vi "Test - Serial Device - Write Pin 1.vi"(8 "error in (no error)":errorcluster, 11 "Module ID":i32) -> (0 "error out":errorcluster, 3 "Pass":bool)   [LabVIEW 2020]
doc: "_____\nCreated using Delacor QMH Event Scripter 5.0.0.112."
uses:
  Libraries/Serial Device/Serial Device.lvlib
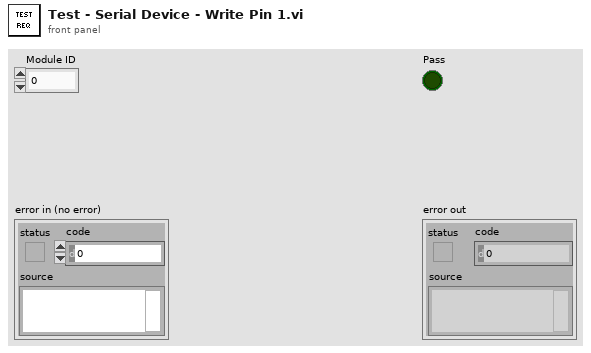
[diagram p1: front panel]
types:
  T1 = typedef "Serial Device.lvlib/Broadcast Events--cluster.ctl" = cluster{"Module Did Init":refnum<user-event>, "Status Updated":refnum<user-event>, "Error Reported":refnum<user-event>, "Module Did Stop":refnum<user-event>, "Update Module Execution Status":refnum<user-event>}
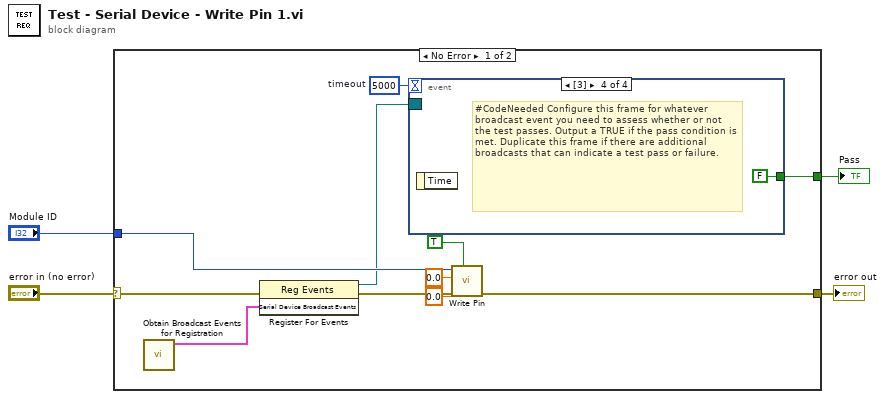
[diagram p0: block diagram]
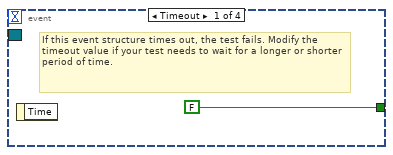
[diagram p2: hidden frame]
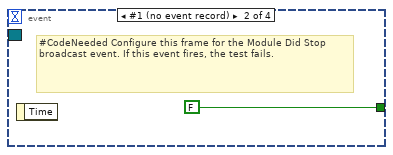
[diagram p3: hidden frame]
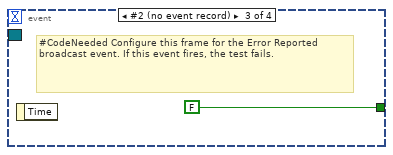
[diagram p4: hidden frame]
diagram:
  n1 = case shown="No Error" "error in (no error)" {
    selector: "error in (no error)" -> [w15 w20]
    tunnel: [w14 w20] -> w3
    tunnel: "Module ID" -> [w13 _]
    tunnel: [w8 _] -> w1
    frame No Error {
      w9 = 5000  # timeout
      n2 = call "Obtain Broadcast Events for Registration.vi"() -> ("Serial Device Broadcast Events"=w11:T1)  [unwired: 9 in, 2 out]
      n3 = register-events(error in=w15, w11) -> (reference out=w10:refnum<event-registration>, error out=w12:errorcluster)  [unwired: 1 in]
      n4 = event shown="[3]" {
        selector: w10 -> [_ _ _ _]
        dyn-events: _ -> [_ _ _ _]
        timeout: w9 -> [_ _ _ _]
        tunnel: [FALSE FALSE FALSE FALSE] -> w8
        event Timeout {
          # "If this event structure times out, the test fails. Modify the timeout value if your test needs to wait for a longer or shorter period of time."
          n5 = event-data() -> ()  [unwired: 1 in, 1 out]
        }
        event #1 (no event record) {
          # "#CodeNeeded Configure this frame for the Module Did Stop broadcast event. If this event fires, the test fails."
          n6 = event-data() -> ()  [unwired: 1 in, 1 out]
        }
        event #2 (no event record) {
          # "#CodeNeeded Configure this frame for the Error Reported broadcast event. If this event fires, the test fails."
          n7 = event-data() -> ()  [unwired: 1 in, 1 out]
        }
        event #3 (no event record) {
          # "#CodeNeeded Configure this frame for whatever broadcast event you need to assess whether or not the test passes. Output a TRUE if the pass condition is met. Duplicate this frame if there are additional broadcasts that can indicate a test pass or failure."
          n8 = event-data() -> ()  [unwired: 1 in, 1 out]
        }
      }
      n9 = call "Write Pin.vi"("Value"=TRUE, "error in (no error)"=w12, "Pin"=0.0, "Port"=0.0, "Module ID"=w13) -> ("error out"=w14:errorcluster)  [unwired: 6 in]
    }
    frame Error {
    }
  }
  "error out" <- w3
  "Pass" <- w1
